vi "FRCts20_WebMethods_ESP_Request.vi"(8 "error in (no error)":errorcluster, 9 "Request":T1, 10 "Return Type":T3="mobile", 11 "httpRequestID":u32) -> (0 "error out":errorcluster, 3 "httpRequestID out":u32)   [LabVIEW 2014, in "FRCts20_WebMethods.lvlib"]
uses:
  FRCts20_WebMethods.lvlib
  Controls/FRCts20_WebMethods_ctl_returntype.ctl
  Backend/source/VI Source/FRCts20_Backend_API/FRCts20_Backend_API_Request.ctl
  Backend/source/VI Source/FRCts20_Backend_API/FRCts20_Backend_API_Status.ctl
  Controls/FRCts20_WebMethods_Globals.vi
  <vilib>/wsapi/subVIs/Set String ESP Variable.vi
  <vilib>/wsapi/subVIs/Set Integer ESP Variable.vi
  <vilib>/wsapi/NI_WebServices.lvlib
  Backend/source/VI Source/FRCts20_Backend_API/FRCts20_Backend_API.lvlib
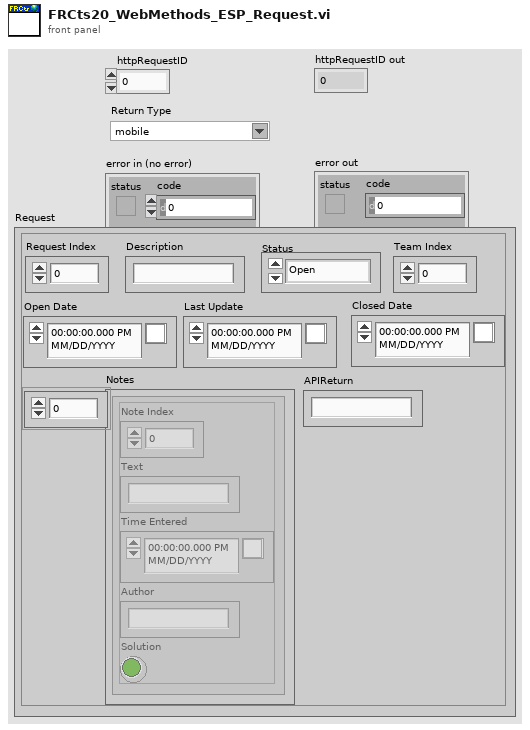
[diagram p1: front panel]
types:
  T1 = typedef "FRCts20_Backend_API.lvlib/FRCts20_Backend_API_Request.ctl" = cluster{"Request Index":u32, "Description":string, "Status":T2, "Open Date":timestamp, "Last Update":timestamp, "Closed Date":timestamp, "Notes":cluster{"Note Index":u32, "Text":string, "Time Entered":timestamp, "Author":string, "Solution":bool}[], "Team Index":u32, "APIReturn":string}
  T2 = typedef "FRCts20_Backend_API.lvlib/FRCts20_Backend_API_Status.ctl" = enum16{"Open", "In Work", "Closed"}
  T3 = typedef "FRCts20_WebMethods.lvlib/FRCts20_WebMethods_ctl_returntype.ctl" = string
  T4 = cluster{"Note Index":u32, "Text":string, "Time Entered":timestamp, "Author":string, "Solution":bool}[]
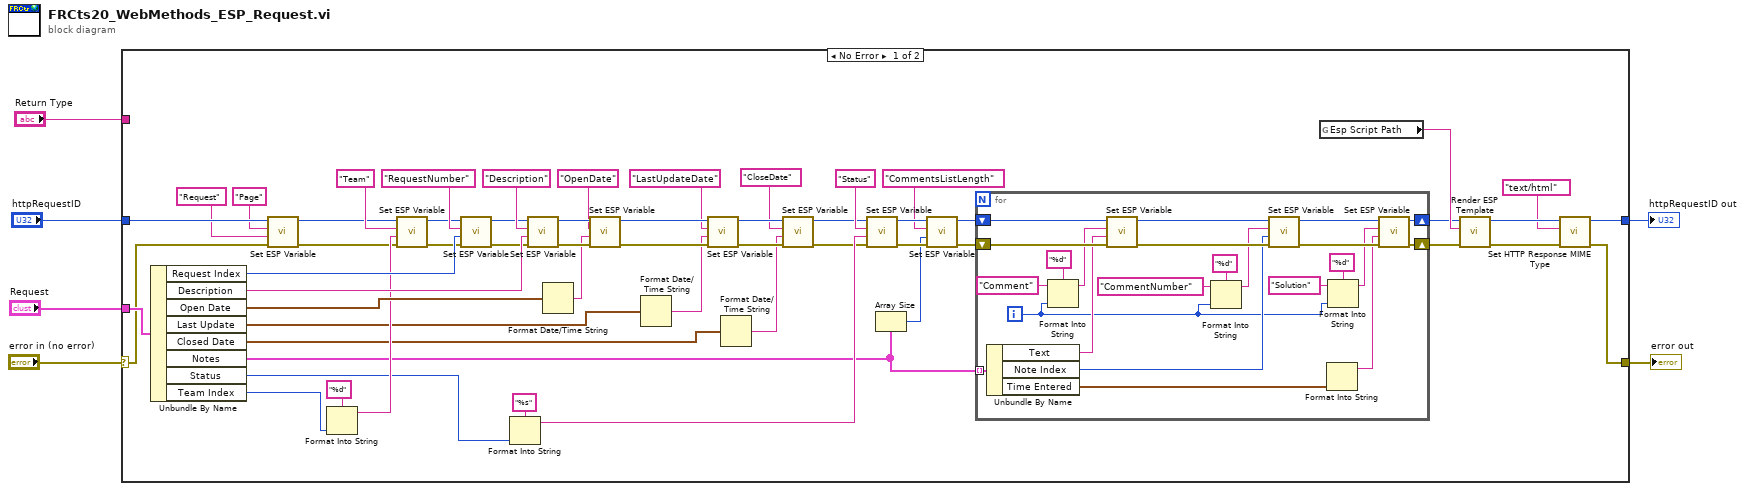
[diagram p0: block diagram]
diagram:
  n1 = case shown="No Error" "error in (no error)" {
    selector: "error in (no error)" -> [w23 w86]
    tunnel: "httpRequestID" -> [w26 w85]
    tunnel: [w59 w85] -> w3
    tunnel: [w58 w86] -> w2
    tunnel: "Return Type" -> [_ _]
    tunnel: "Request" -> [w35 _]
    frame No Error {
      n2 = Unbundle By Name(w35) -> ("Request Index"=w47:u32, "Description"=w54:string, "Open Date"=w43:timestamp, "Last Update"=w18:timestamp, "Closed Date"=w10:timestamp, "Notes"=w19:T4, "Status"=w20:T2, "Team Index"=w21:u32)
      n3 = call-poly <vilib>:"Set ESP Variable.vi"("error in (no error)"=w23, "value"="Request", "key"="Page", "httpRequestID"=w26) -> ("error out"=w28:errorcluster, "httpRequestID out"=w27:u32)  [unwired: 6 in]
      n4 = Format Into String(format string="%d", w21) -> (resulting string=w31:string)  [unwired: 2 in, 1 out]
      n5 = call-poly <vilib>:"Set ESP Variable.vi"("error in (no error)"=w28, "value"=w31, "key"="Team", "httpRequestID"=w27) -> ("error out"=w32:errorcluster, "httpRequestID out"=w33:u32)  [unwired: 6 in]
      n6 = call-poly <vilib>:"Set ESP Variable.vi"("error in (no error)"=w32, "value"=w47, "key"="RequestNumber", "httpRequestID"=w33) -> ("error out"=w53:errorcluster, "httpRequestID out"=w52:u32)  [unwired: 6 in]
      n7 = Format Into String(format string="%s", w20) -> (resulting string=w50:string)  [unwired: 2 in, 1 out]
      n8 = call-poly <vilib>:"Set ESP Variable.vi"("error in (no error)"=w53, "value"=w54, "key"="Description", "httpRequestID"=w52) -> ("error out"=w46:errorcluster, "httpRequestID out"=w45:u32)  [unwired: 6 in]
      n9 = Format Date/Time String(seconds (now)=w43) -> (date/time string=w42:string)  [unwired: 2 in]
      n10 = call-poly <vilib>:"Set ESP Variable.vi"("error in (no error)"=w46, "value"=w42, "key"="OpenDate", "httpRequestID"=w45) -> ("error out"=w22:errorcluster, "httpRequestID out"=w41:u32)  [unwired: 6 in]
      n11 = Format Date/Time String(seconds (now)=w18) -> (date/time string=w16:string)  [unwired: 2 in]
      n12 = call-poly <vilib>:"Set ESP Variable.vi"("error in (no error)"=w22, "value"=w16, "key"="LastUpdateDate", "httpRequestID"=w41) -> ("error out"=w15:errorcluster, "httpRequestID out"=w14:u32)  [unwired: 6 in]
      n13 = Format Date/Time String(seconds (now)=w10) -> (date/time string=w9:string)  [unwired: 2 in]
      n14 = call-poly <vilib>:"Set ESP Variable.vi"("error in (no error)"=w15, "value"=w9, "key"="CloseDate", "httpRequestID"=w14) -> ("error out"=w12:errorcluster, "httpRequestID out"=w13:u32)  [unwired: 6 in]
      n15 = call-poly <vilib>:"Set ESP Variable.vi"("error in (no error)"=w12, "value"=w50, "key"="Status", "httpRequestID"=w13) -> ("error out"=w49:errorcluster, "httpRequestID out"=w48:u32)  [unwired: 6 in]
      n16 = Array Size(array=w19) -> (size(s)=w39:i32)
      n17 = call-poly <vilib>:"Set ESP Variable.vi"("error in (no error)"=w49, "value"=w39, "key"="CommentsListLength", "httpRequestID"=w48) -> ("error out"=w40:errorcluster, "httpRequestID out"=w36:u32)  [unwired: 6 in]
      n18 = for {
        shift-right: [w70] -> w37
        shift-left: w40 -> [w84]
        tunnel: w19 -> [w79] mode=indexing
        shift-right: [w69] -> w8
        shift-left: w36 -> [w80]
        i -> [w65]
        n19 = Unbundle By Name(w79) -> ("Text"=w78:string, "Note Index"=w72:u32, "Time Entered"=w63:timestamp)
        n20 = Format Into String(format string="%d", initial string="Comment", w65) -> (resulting string=w82:string)  [unwired: 1 in, 1 out]
        n21 = call-poly <vilib>:"Set ESP Variable.vi"("error in (no error)"=w84, "value"=w78, "key"=w82, "httpRequestID"=w80) -> ("error out"=w77:errorcluster, "httpRequestID out"=w76:u32)  [unwired: 6 in]
        n22 = Format Into String(format string="%d", initial string="CommentNumber", w65) -> (resulting string=w73:string)  [unwired: 1 in, 1 out]
        n23 = call-poly <vilib>:"Set ESP Variable.vi"("error in (no error)"=w77, "value"=w72, "key"=w73, "httpRequestID"=w76) -> ("error out"=w68:errorcluster, "httpRequestID out"=w71:u32)  [unwired: 6 in]
        n24 = Format Into String(w63) -> (resulting string=w62:string)  [unwired: 3 in, 1 out]
        n25 = Format Into String(format string="%d", initial string="Solution", w65) -> (resulting string=w64:string)  [unwired: 1 in, 1 out]
        n26 = call-poly <vilib>:"Set ESP Variable.vi"("error in (no error)"=w68, "value"=w62, "key"=w64, "httpRequestID"=w71) -> ("error out"=w70:errorcluster, "httpRequestID out"=w69:u32)  [unwired: 6 in]
      }
      n27 = global read "FRCts20_WebMethods_Globals.vi" "Esp Script Path"() -> (w34:string)
      n28 = call <vilib>:"Render ESP Template.vi"("error in (no error)"=w37, "espName"=w34, "httpRequestID"=w8) -> ("error out"=w60:errorcluster, "httpRequestID out"=w61:u32)  [unwired: 7 in]
      n29 = call <vilib>:"Set HTTP Response MIME Type.vi"("error in (no error)"=w60, "MIME type (text/html)"="text/html", "httpRequestID"=w61) -> ("error out"=w58:errorcluster, "httpRequestID out"=w59:u32)  [unwired: 7 in]
    }
    frame Error {
    }
  }
  "httpRequestID out" <- w3
  "error out" <- w2
